vi "Pacemaker ASIC Test_Warning Globals.vi"() -> ()   [LabVIEW 2012]
panel:
  out "new warnings":string
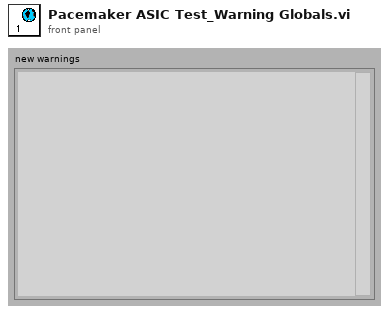
[diagram p1: front panel]
diagram:
